vi "fire&temp&smoke&level sensors with LabView.vi"() -> ()   [LabVIEW 2020]
panel:
  in  "Tab Control":enum32{"Page 1", "Page 2", "Page 3"}(tab)
  out "F_lv2":dbl(slide) scale=0.0..1200.0 scale format="%#_6f"
  out "F_lev 2":dbl
  out "fuel_level METER":dbl(knob) scale=0.0..1200.0
  out "leve; Indicator 3":bool
  out "Temperature":dbl(slide) scale=0.0..100.0
  out "TEMP":dbl(graph)
  out "temp":dbl
  in  "Table Control":string[][](table)
  out "FIRE Indicator":bool
  out "FIRE 2":bool
  out "smoke Indicator 1":bool
  out "SMOKE 2":bool
  out "SMOKE METER":dbl(knob) scale=0.0..1.0
  out "FIRE METER":dbl(knob) scale=0.0..1.0
  out "FIRE":i32(graph)
  out "SMOKE":i32(graph)
  out "FIRE Indicator2":bool
  out "smoke Indicator 2":bool
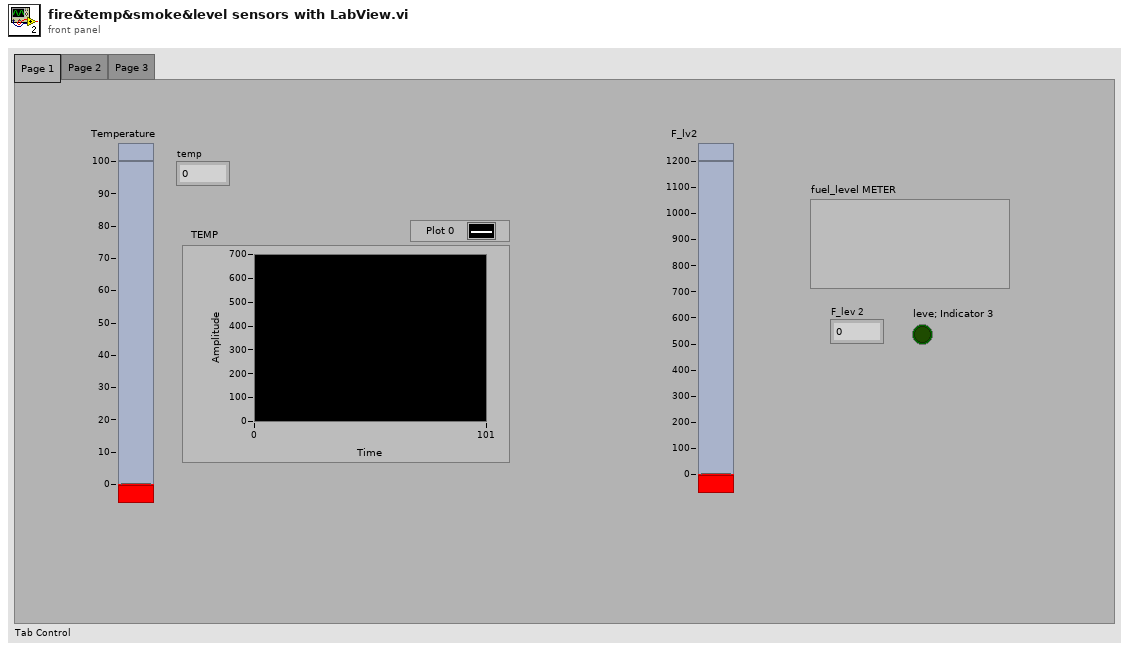
[diagram p1: front panel]
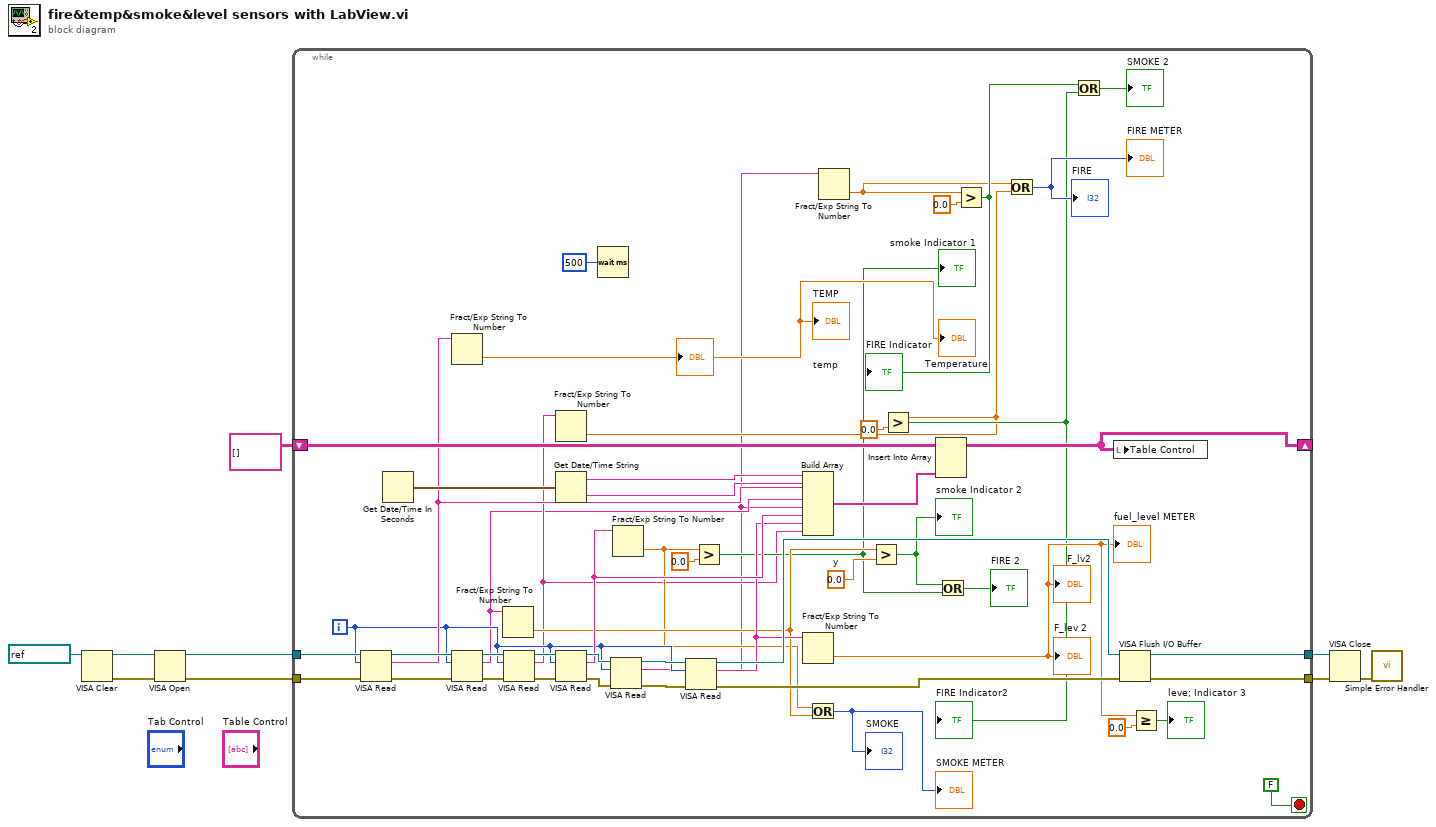
[diagram p0: block diagram]
diagram:
  n1 = VISA Clear(VISA resource name=refnum<visa-resource-name> "COM2") -> (VISA resource name out=w9:refnum<visa-resource-name>, error out=w8:errorcluster)  [unwired: 1 in]
  n2 = VISA Open(error in (no error)=w8, VISA resource name=w9) -> (VISA resource name=w7:refnum<visa-resource-name>, error out=w6:errorcluster)  [unwired: 3 in]
  n3 = while {
    shift-right: [w24] -> _
    shift-left: string[][] [] -> [w51]
    tunnel: w7 -> [w59]
    tunnel: w6 -> [w58]
    tunnel: [w53] -> w5
    tunnel: [w52] -> w4
    i -> [w29]
    stop <- FALSE ("stop") stop-if-true
    w43 = 0.0  # y
    n4 = VISA Read(VISA resource name=w59, byte count=w29, error in (no error)=w58) -> (VISA resource name out=w57:refnum<visa-resource-name>, read buffer=w47:string, error out=w56:errorcluster)  [unwired: 1 out]
    n5 = Get Date/Time In Seconds() -> (seconds since 1Jan1904=w50:timestamp)
    n6 = Fract/Exp String To Number(string=w47) -> (number=→"Temperature" →"TEMP" →"temp":dbl)  [unwired: 3 in, 1 out]
    n7 = VISA Read(VISA resource name=w57, byte count=w29, error in (no error)=w56) -> (VISA resource name out=w55:refnum<visa-resource-name>, read buffer=w11:string, error out=w54:errorcluster)  [unwired: 1 out]
    n8 = Fract/Exp String To Number(string=w11) -> (number=w17:dbl)  [unwired: 3 in, 1 out]
    n9 = VISA Read(VISA resource name=w55, byte count=w29, error in (no error)=w54) -> (VISA resource name out=w36:refnum<visa-resource-name>, read buffer=w13:string, error out=w35:errorcluster)  [unwired: 1 out]
    n10 = Fract/Exp String To Number(string=w13) -> (number=w15:dbl)  [unwired: 3 in, 1 out]
    n11 = Get Date/Time String(seconds (now)=w50) -> (date string=w49:string, time string=w48:string)  [unwired: 2 in]
    n12 = VISA Read(VISA resource name=w36, byte count=w29, error in (no error)=w35) -> (VISA resource name out=w38:refnum<visa-resource-name>, read buffer=w30:string, error out=w37:errorcluster)  [unwired: 1 out]
    n13 = Wait (ms)(milliseconds to wait=u32 500) -> ()  [unwired: 1 out]
    n14 = VISA Read(VISA resource name=w38, byte count=w29, error in (no error)=w37) -> (VISA resource name out=w34:refnum<visa-resource-name>, read buffer=w10:string, error out=w33:errorcluster)  [unwired: 1 out]
    n15 = Fract/Exp String To Number(string=w30) -> (number=w16:dbl)  [unwired: 3 in, 1 out]
    n16 = VISA Read(VISA resource name=w34, byte count=w29, error in (no error)=w33) -> (VISA resource name out=w32:refnum<visa-resource-name>, read buffer=w21:string, error out=w31:errorcluster)  [unwired: 1 out]
    n17 = Greater?(x=w16, y=0.0) -> (0:w14:bool)
    "smoke Indicator 1" <- w14
    n18 = Build Array "Build Array"(w49, w48, w47, w11, w10, w30, w21, w13) -> (w44:string[])
    n19 = Fract/Exp String To Number(string=w21) -> (number=w27:dbl)  [unwired: 3 in, 1 out]
    "F_lv2" <- w27
    "F_lev 2" <- w27
    "fuel_level METER" <- w27
    n20 = Or(x=w16, y=w17) -> (x .or. y?=→"SMOKE" →"SMOKE METER":i32)
    n21 = Fract/Exp String To Number(string=w10) -> (number=w39:dbl)  [unwired: 3 in, 1 out]
    n22 = Greater?(x=w17, y=w43) -> (0:w18:bool)
    "smoke Indicator 2" <- w18
    n23 = Greater?(x=w15, y=0.0) -> (0:w19:bool)
    "FIRE Indicator2" <- w19
    n24 = Insert Into Array "Insert Into Array"(array=w51, new element=w44) -> (w24:string[][])  [unwired: 2 in]
    n25 = Or(x=w18, y=w14) -> (x .or. y?=→"FIRE 2":bool)
    n26 = Greater?(x=w39, y=0.0) -> (0:w41:bool)
    "FIRE Indicator" <- w41
    n27 = Or(x=w39, y=w15) -> (x .or. y?=→"FIRE" →"FIRE METER":i32)
    n28 = Or(x=w41, y=w19) -> (x .or. y?=→"SMOKE 2":bool)
    n29 = local write "Table Control"(w24) -> ()
    n30 = VISA Flush I/O Buffer(VISA resource name=w32, error in (no error)=w31) -> (VISA resource name out=w53:refnum<visa-resource-name>, error out=w52:errorcluster)  [unwired: 1 in]
    n31 = Greater Or Equal?(x=w27, y=0.0) -> (x >= y?=→"leve; Indicator 3":bool)
  }
  n32 = VISA Close(VISA resource name=w5, error in (no error)=w4) -> (error out=w3:errorcluster)
  n33 = call <vilib>:"Simple Error Handler.vi"("error in (no error)"=w3) -> ()  [unwired: 4 in, 5 out]
